vi "run.vi"(8 "results reporter":refnum<class "results reporter.lvclass">, 9 "execution system":T1=enum."standard", 10 "thread pool":refnum<class "thread pool.lvclass">, 11 "batch task in":refnum<class "batch task.lvclass">) -> (2 "result":refnum<class "result.lvclass">, 3 "batch task out":refnum<class "batch task.lvclass">)   [LabVIEW 2014, in "batch task.lvclass"]
uses:
  batch task.lvclass
  result/result.lvclass
  dispatcher/thread pool.lvclass
  dispatcher/execution system.ctl
  results reporter/results reporter.lvclass
  batch task.lvclass/batch task.ctl
  standard reporters/queue reporter/queue reporter.lvclass
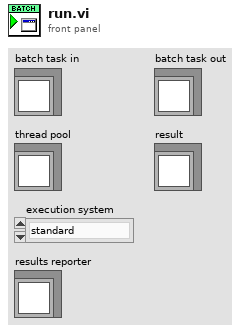
[diagram p1: front panel]
types:
  T1 = typedef "thread pool.lvclass/execution system.ctl" = enum32{"user interface", "standard", "instrument i/o", "data acquisition", "other 1", "other 2"}
  T2 = typedef "batch task.lvclass/reporting type.ctl" = enum16{"return immediately", "wait on all"}
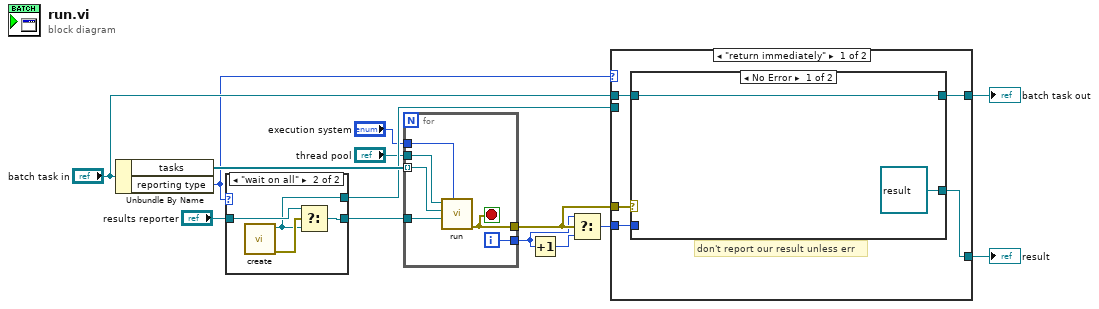
[diagram p0: block diagram]
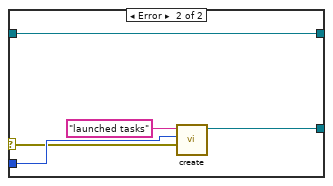
[diagram p2: hidden frame]
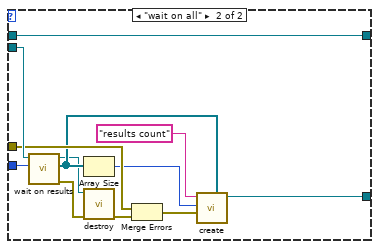
[diagram p3: hidden frame]
diagram:
  n1 = Unbundle By Name("batch task in") -> ("tasks"=w13:refnum<class "task.lvclass">[], "reporting type"=w11:T2)
  n2 = case shown="\"wait on all\"" w11 {
    tunnel: [w15 w17] -> w12
    tunnel: "results reporter" -> [w15 w18]
    tunnel: [_ w16] -> w8
    frame "return immediately" {
    }
    frame "wait on all" {
      n3 = call "create.vi"() -> ("error out"=w19:errorcluster, "queue reporter out"=w16:refnum<class "queue reporter.lvclass">)  [unwired: 10 in]
      n4 = Select(t=w18, s=w19, f=w16) -> (s? t:f=w17:refnum<class "results reporter.lvclass">)
    }
  }
  n5 = for {
    tunnel: w13 -> [w22] mode=indexing
    tunnel: w12 -> [w21]
    tunnel: [w25] -> w6
    tunnel: [w24] -> w5
    tunnel: "execution system" -> [w20]
    tunnel: "thread pool" -> [w23]
    i -> [w24]
    stop <- w25 stop-if-true
    n6 = call "run.vi"("execution system"=w20, "results reporter"=w21, "task"=w22, "thread pool in"=w23) -> ("error out"=w25:errorcluster)  [unwired: 6 in, 1 out]
  }
  n7 = Increment(x=w5) -> (x+1=w4:i32)
  n8 = Select(t=w5, s=w6, f=w4) -> (s? t:f=w7:i32)
  n9 = case shown="\"return immediately\"" w11 {
    tunnel: [w29 w49] -> w10
    tunnel: "batch task in" -> [w30 w49]
    tunnel: [w28 w45] -> w9
    tunnel: w8 -> [_ w48]
    tunnel: w6 -> [w27 w44]
    tunnel: w7 -> [w26 w47]
    frame "return immediately" {
      # "don't report our result unless err"
      n10 = case shown="No Error" w27 {
        selector: w27 -> [_ w34]
        tunnel: w30 -> [w32 w37]
        tunnel: [w32 w37] -> w29
        tunnel: [refnum<class "result.lvclass"> refnum ("result") w36] -> w28
        tunnel: w26 -> [_ w35]
        frame No Error {
        }
        frame Error {
          n11 = call "create.vi"("error"=w34, "data"=w35, "data ID"="launched tasks") -> ("result out"=w36:refnum<class "result.lvclass">)  [unwired: 8 in]
        }
      }
    }
    frame "wait on all" {
      n12 = call "wait on results.vi"("count"=w47, "queue reporter in"=w48) -> ("error out"=w46:errorcluster, "results"=w40:refnum<class "result.lvclass">[], "queue reporter out"=w38:refnum<class "queue reporter.lvclass">)  [unwired: 7 in]
      n13 = Array Size(array=w40) -> (size(s)=w42:i32)
      n14 = call-dynamic "destroy.vi"("error in"=w46, "queue reporter in"=w38) -> ("error out"=w39:errorcluster)  [unwired: 9 in]
      n15 = Merge Errors(w44, w39) -> (w43:errorcluster)
      n16 = call "create.vi"("subresults"=w40, "error"=w43, "data"=w42, "data ID"="results count") -> ("result out"=w45:refnum<class "result.lvclass">)  [unwired: 7 in]
    }
  }
  "result" <- w9
  "batch task out" <- w10
